vi "CryoCon Parse SensorType.vi"(1 "String Read":string) -> (0 "Sensor Type 2":T1)   [LabVIEW 2019]
uses:
  Sub Controls/CryoCon Sensor Type.ctl
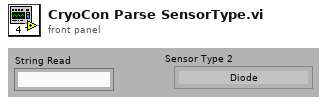
[diagram p1: front panel]
types:
  T1 = typedef "CryoCon Sensor Type.ctl" = enum16{"Diode", "AC Resistance", "DC Resistance 3.1 k½", "DC Resistance 312 ½", "DC Resistance 625 ½"}
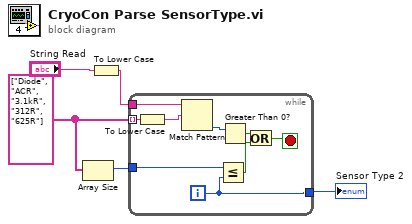
[diagram p0: block diagram]
diagram:
  w2 = string[] ["Diode", "ACR", "3.1kR", "312R", "625R"]
  n1 = Array Size(array=w2) -> (size(s)=w3:i32)
  n2 = To Lower Case(string="String Read") -> (all lower case string=w1:string)
  n3 = while {
    tunnel: w2 -> [w13] mode=indexing
    tunnel: w1 -> [w14]
    tunnel: [w8] -> w5
    tunnel: w3 -> [w7]
    i -> [w8]
    stop <- w10 stop-if-true
    n4 = To Lower Case(string=w13) -> (all lower case string=w6:string)
    n5 = Match Pattern(string=w14, regular expression=w6) -> (offset past match=w12:i32)  [unwired: 1 in, 3 out]
    n6 = Less Or Equal?(x=w7, y=w8) -> (x <= y?=w9:bool)
    n7 = Greater Than 0?(x=w12) -> (x > 0?=w11:bool)
    n8 = Or(x=w11, y=w9) -> (x .or. y?=w10:bool)
  }
  "Sensor Type 2" <- w5
